vi "Google Spreadsheet String.vi"(9 "Array Value":string[](array[string])=["11", "22", "44", "66", "77", "99", "1111"], 11 "Array Index":string[](array[string])=["1", "2", "4", "6", "7", "9", "11"]) -> (1 "size(s) 2":i32, 2 "size(s)":i32, 3 "Output string":string)   [LabVIEW 2011]
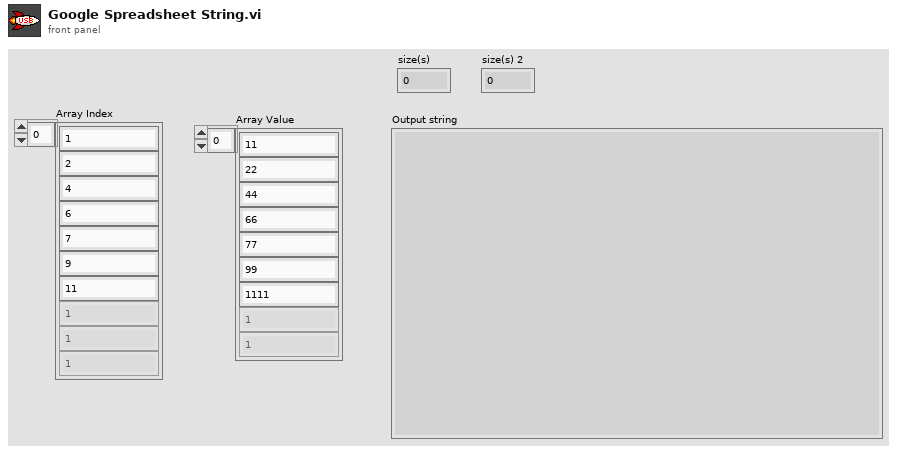
[diagram p1: front panel]
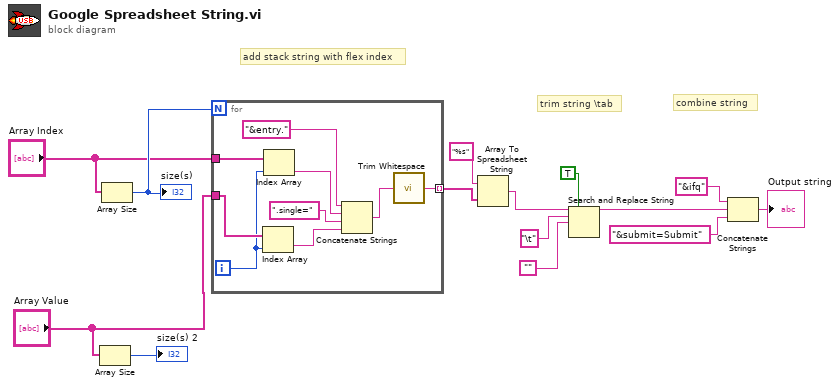
[diagram p0: block diagram]
diagram:
  # "add stack string with flex index"
  # "combine string"
  # "trim string \\tab"
  n1 = Array Size(array="Array Value") -> (size(s)=→"size(s) 2":i32)
  n2 = Array Size(array="Array Index") -> (size(s)=w14:i32)
  "size(s)" <- w14
  n3 = for {
    N: w14 -> [_]
    tunnel: "Array Value" -> [w23]
    tunnel: "Array Index" -> [w18]
    tunnel: [w15] -> w9 mode=indexing
    i -> [w19]
    n4 = Index Array(array=w23, index=w19) -> (element=w22:string)
    n5 = Index Array(array=w18, index=w19) -> (element=w17:string)
    n6 = Concatenate Strings("&entry.", w17, ".single=", w22) -> (w16:string)
    n7 = call <vilib>:"Trim Whitespace.vi"("string"=w16) -> ("trimmed string"=w15:string)  [unwired: 1 in]
  }
  n8 = Array To Spreadsheet String(array=w9, 3:"%s" ("format string")) -> (spreadsheet string=w7:string)  [unwired: 1 in]
  n9 = Search and Replace String(replace all?=TRUE ("replace all? (F)"), input string=w7, search string="\t", replace string="") -> (result string=w3:string)  [unwired: 4 in, 3 out]
  n10 = Concatenate Strings("&ifq" ("string"), w3, "&submit=Submit" ("string")) -> (→"Output string":string)
